vi "ULx Read (Digital 2D Bool NChan 1Samp NLine).vi"(0 "task in":refnum<k24>, 9 "timeout":dbl=10.0 format="%_4g", 11 "error in":errorcluster) -> (4 "task out":refnum<k24>, 6 "data":bool[][](array[boolean]), 15 "error out":errorcluster)   [LabVIEW 2020]
doc: "Reads a single sample that contains Boolean values from each channel in a task that contains one or more digital input channels. Each channel can contain multiple digital lines."
uses:
  C:/Users/William/Documents/LV 2020 builds/LeaktestDAQ/Source-v33/ULx_LV.dll
  ULx_LV.dll
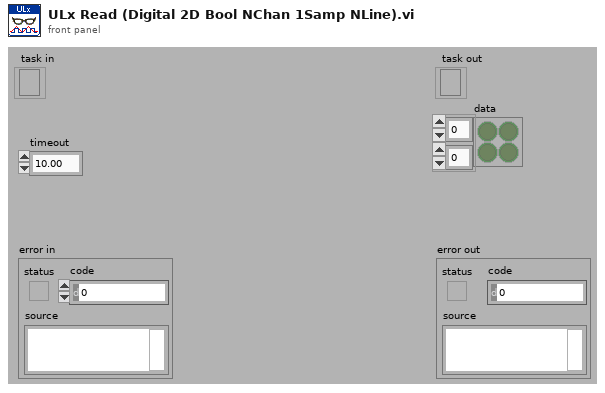
[diagram p1: front panel]
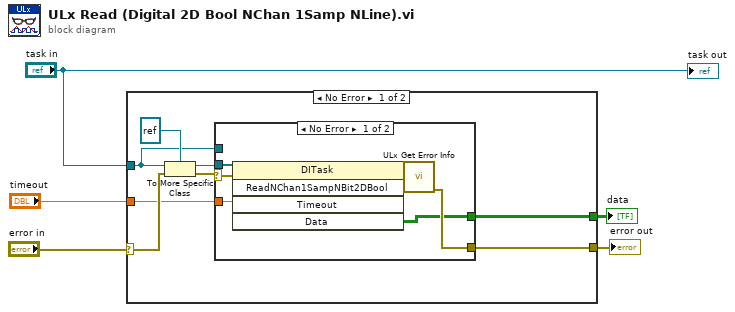
[diagram p0: block diagram]
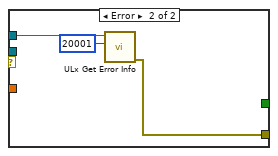
[diagram p2: hidden frame]
diagram:
  n1 = case shown="No Error" "error in" {
    selector: "error in" -> [w13 w25]
    tunnel: "task in" -> [w6 _]
    tunnel: "timeout" -> [w9 _]
    tunnel: [w8 w25] -> w3
    tunnel: [w7 _] -> w1
    frame No Error {
      n2 = To More Specific Class(target class=refnum<k24> refnum, reference=w6, error in=w13) -> (specific class reference=w10:refnum<k24>, error out=w11:errorcluster)
      n3 = case shown="No Error" w11 {
        selector: w11 -> [w20 _]
        tunnel: w10 -> [w21 _]
        tunnel: w9 -> [w16 _]
        tunnel: [w17 w22] -> w8
        tunnel: [w15 _] -> w7
        tunnel: w6 -> [_ w24]
        frame No Error {
          n4 = invoke class="DITask" method="ReadNChan1SampNBit2DBool"(reference=w21, error in=w20, "Timeout"=w16) -> (reference out=w18:refnum<k24>, error out=w19:errorcluster, "ReadNChan1SampNBit2DBool"=w14:i32, "Data"=w15:bool[][])  [unwired: 2 in, 1 out]
          n5 = call "ULx Get Error Info.vi"("error in"=w19, "ErrorCode"=w14, "task in"=w18) -> ("error out"=w17:errorcluster)  [unwired: 8 in]
        }
        frame Error {
          n6 = call "ULx Get Error Info.vi"("ErrorCode"=20001, "task in"=w24) -> ("error out"=w22:errorcluster)  [unwired: 9 in]
        }
      }
    }
    frame Error {
    }
  }
  "error out" <- w3
  "data" <- w1
  "task out" <- "task in"
